vi "PYTHON New Session__ogtk.vi"(4 "error in (no error)":errorcluster) -> (0 "error out":errorcluster, 3 "Python Session":T1)   [LabVIEW 2010]
doc: "This function makes sure the Python shared library is properly loaded and then creates a session context which is used to store the input and output variables, the human readable and compiled script, and any error state information which might occur during execution on this session refnum."
uses:
  Python Session Refnum__ogtk.ctl
  lvpython.dll
panel:
  # "PYTHON New Session.vi\n\nCreate a new session context to be used for script operations\n\nCopyright (C) 2002 Rolf Kalbermatter rolf.kalbermatter@citeng.com\nCopyright (C) 2002 James Kring jim@jimkring.com\n\nPlease visit http://www.OpenG.org to learn about the\nOpen Source LabVIEW software movement.\n\nThis library is free software; you can redistribute it and/or\nmodify it under the terms of the GNU Lesser General Public\nLicense as published by the Free Software Foundation; either\nversion 2.1 of the License, or (at your option) any later version.\nThis library is distributed in the hope that it will be useful,\nbut WITHOUT ANY WARRANTY; without even the implied warranty of\nMERCHANTABILITY or FITNESS FOR A PARTICULAR PURPOSE. See the GNU\nLesser General Public License for more details.\nYou should have received a copy of the GNU Lesser General Public\nLicense along with this library; if not, write to the Free Software\nFoundation, Inc., 59 Temple Place, Suite 330, Boston, MA 02111-1307 USA"
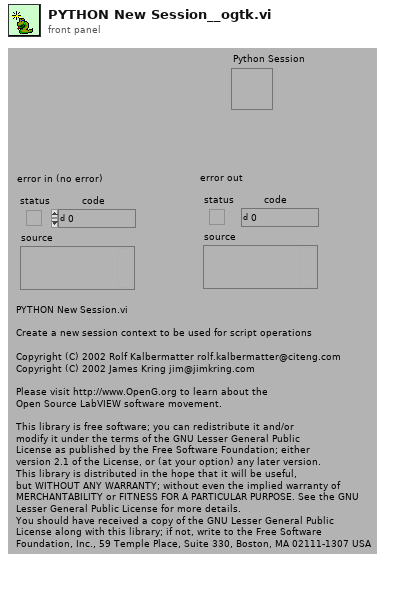
[diagram p1: front panel]
types:
  T1 = typedef "Python Session Refnum__ogtk.ctl" = refnum<k1>
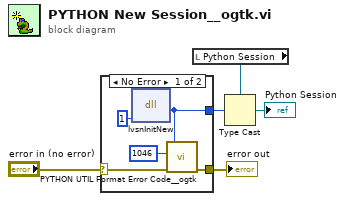
[diagram p0: block diagram]
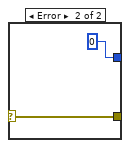
[diagram p2: hidden frame]
diagram:
  n1 = case shown="No Error" "error in (no error)" {
    selector: "error in (no error)" -> [w9 w12]
    tunnel: [w8 u32 0 ("session")] -> w2
    tunnel: [w6 w12] -> w4
    frame No Error {
      n2 = dll-call lib="C:/UdeM/BonOMM-10/LabVIEW/labpython/lvpython.*" fn="lvsnInitNew"(1 ("Input Value")) -> (w8:u32)  [unwired: 4 in, 2 out]
      n3 = call "PYTHON UTIL Format Error Code__ogtk.vi"("error in (no error)"=w9, "code"=1046, "Bool32"=w8) -> ("error out"=w6:errorcluster)  [unwired: 4 in]
    }
    frame Error {
    }
  }
  "error out" <- w4
  n4 = local read "Python Session"() -> (w1:T1)
  n5 = Type Cast(type=w1, x=w2) -> (*(type *) &x=→"Python Session":T1)
